vi "Get State.vi"(8 "error in (no error)":errorcluster, 11 "Fluke 1586A Driver in":refnum<class "Fluke 1586A Driver.lvclass">) -> (0 "error out":errorcluster, 1 "Data ready":bool, 2 "Armed":bool, 3 "Fluke 1586A Driver out":refnum<class "Fluke 1586A Driver.lvclass">, 4 "Availiable Samples":u32, 5 "Finished":bool)   [LabVIEW 2021, in "Fluke 1586A Driver.lvclass"]
uses:
  Fluke 1586A Driver.lvclass
  C:/GitHub/NHMFL_Core/Libraries/Instruments/VISA Instrument/VISA Instrument.lvclass
  VISA Instrument/VISA Instrument.lvclass/VISA Instrument.ctl
  VISA Instrument/Read VISA resource.vi
  VISA Instrument/Write VISA resource.vi
  GPIB/VISA  Send Receive.vi
  Simple VISA Reader/Simple VISA Reader Driver.lvclass
panel:
  out "Status":i32 format="%b"
  out "data string out":string
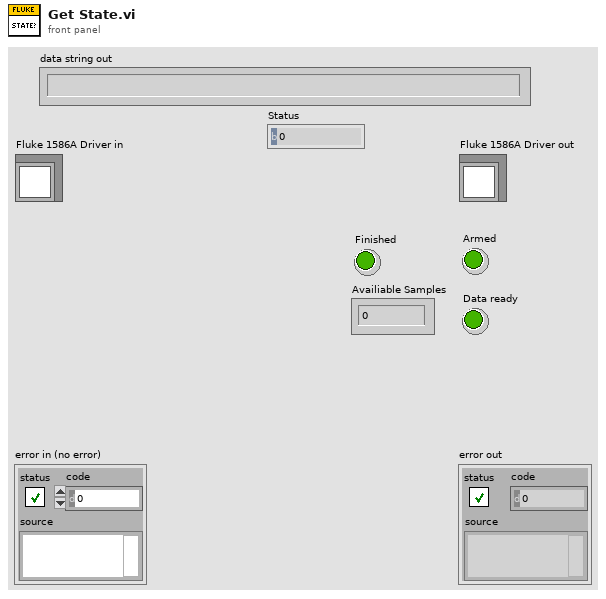
[diagram p1: front panel]
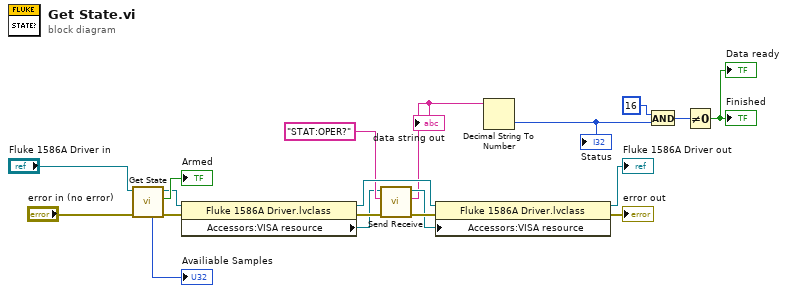
[diagram p0: block diagram]
diagram:
  n1 = call-parent "Get State.vi"("error in (no error)"="error in (no error)", "Instrument Driver in"="Fluke 1586A Driver in") -> ("error out"=w7:errorcluster, "Armed"=→"Armed":bool, "Instrument Driver out"=w9:refnum<class "Fluke 1586A Driver.lvclass">, "Availiable Samples"=→"Availiable Samples":u32)  [unwired: 4 in, 2 out]
  n2 = property class="Fluke 1586A Driver.lvclass"(reference=w9, error in=w7) -> (reference out=w13:refnum<class "Fluke 1586A Driver.lvclass">, error out=w11:errorcluster, "Accessors:VISA resource"=w10:refnum<visa-resource-name>)
  n3 = call-poly "Send Receive.vi"("error in (no error)"=w11, "data string in"="STAT:OPER?", "VISA Resource Name"=w10) -> ("error out"=w15:errorcluster, "data string out"=w5:string, "VISA Resource Name Out"=w14:refnum<visa-resource-name>)  [unwired: 6 in]
  "data string out" <- w5
  n4 = property class="Fluke 1586A Driver.lvclass"(reference=w13, error in=w15, "Accessors:VISA resource"=w14) -> (reference out=→"Fluke 1586A Driver out":refnum<class "Fluke 1586A Driver.lvclass">, error out=→"error out":errorcluster)
  n5 = Decimal String To Number(string=w5) -> (number=w4:i32)  [unwired: 2 in, 1 out]
  "Status" <- w4
  n6 = And(x=16, y=w4) -> (x .and. y?=w2:i32)
  n7 = Not Equal To 0?(x=w2) -> (x != 0?=→"Finished" →"Data ready":bool)
